vi "TestIniLib.vi"() -> ()   [LabVIEW 2014]
uses:
  <vilib>/Utility/config.llb/Config Data RefNum.ctl
  <vilib>/Utility/error.llb/Error Cluster From Error Code.vi
  <vilib>/ErrorRing/Error Ring.xnode
  <vilib>/Utility/config.llb/NI_LVConfig.lvlib
  <userlib>/NIST/NISTErrorLib/NISTErrorLib.lvlib
  Ini_lib.lvlib
panel:
  in  "btnStop":bool
  out "ErrorArray Out":errorcluster[](array[cluster])
  in  "Cluster 3":cluster{"This Array":dbl[]}={"This Array"=[1.0, 2.0, 3.0]}
  in  "Cluster 2":cluster{"This Boolean":bool, "That Path":path}
  in  "Cluster 1":cluster{"This String":string, "That Number":dbl}
  in  "Table 3":string[][](table)
  in  "Table 2":string[][](table)
  in  "Table 1":string[][](table)
  in  "Ring 3":u16(ring) items=["Mod3.Plugin1", "Mod3.Plugin2", "Mod3.Plugin3"]
  in  "Ring 2":u16(ring) items=["Mod2.Plugin1", "Mod2.Plugin2", "Mod2.Plugin3"]
  in  "Ring 1":u16(ring) items=["Mod1.Plugin1", "Mod1.Plugin2", "Mod1.Plugin3"]
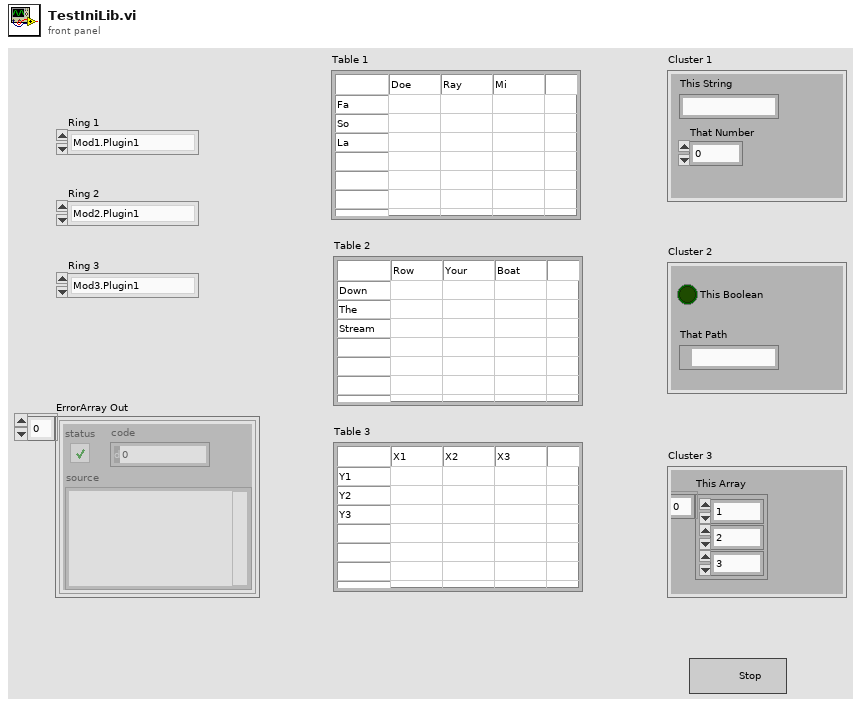
[diagram p1: front panel]
types:
  T1 = cluster{"Ring 1":refnum<vi>, "Table 1":refnum<vi>, "Cluster 1":refnum<vi>, "Ring 2":refnum<vi>, "Table 2":refnum<vi>, "Cluster 2":refnum<vi>, "Ring 3":refnum<vi>, "Table 3":refnum<vi>, "Cluster 3":refnum<vi>}
  T2 = typedef "NI_LVConfig.lvlib/Config Data RefNum.ctl" = refnum<k1>
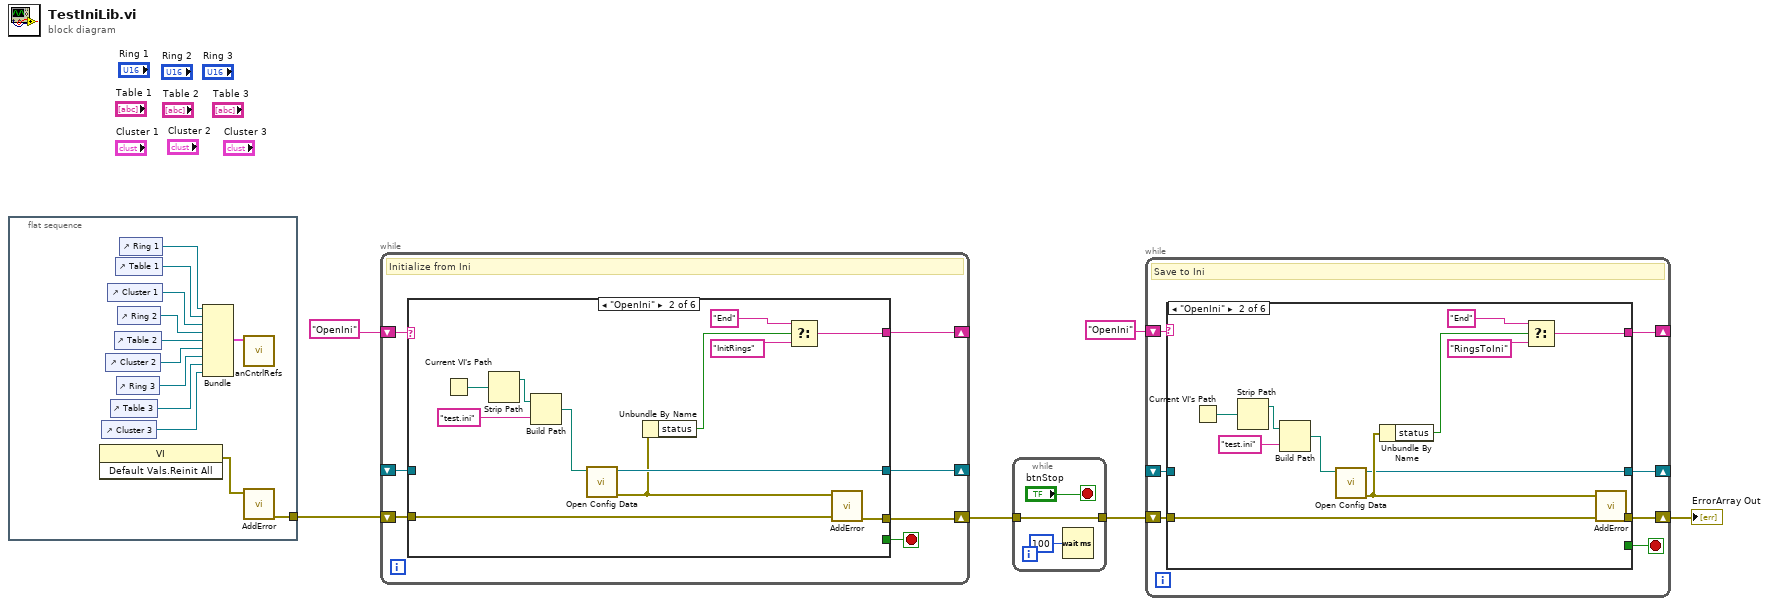
[diagram p0: block diagram]
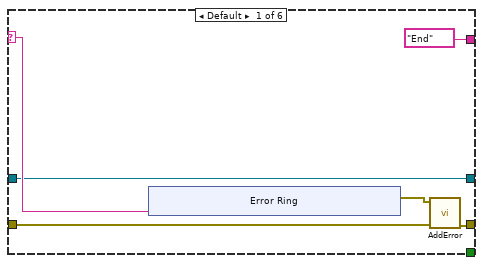
[diagram p2: hidden frame]
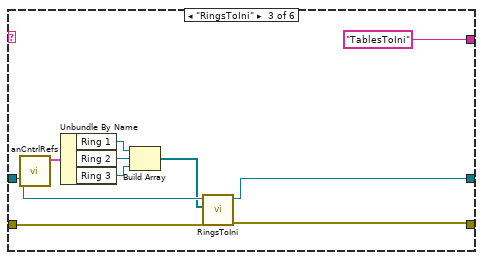
[diagram p3: hidden frame]
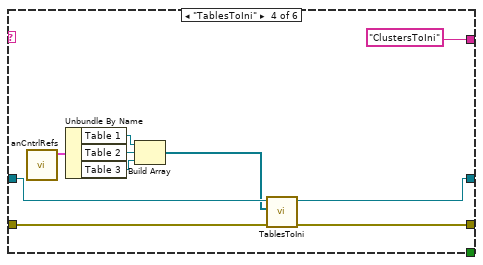
[diagram p4: hidden frame]
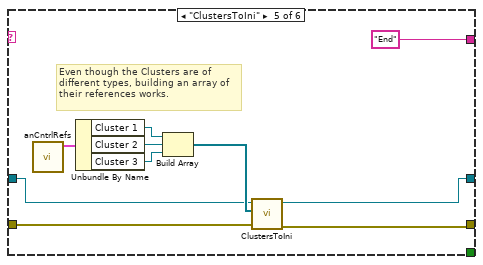
[diagram p5: hidden frame]
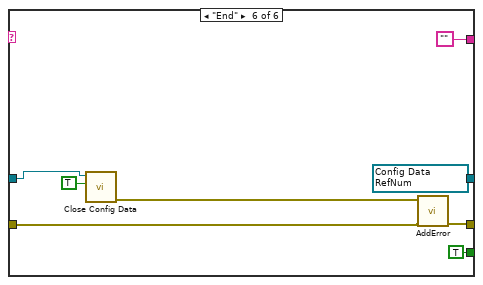
[diagram p6: hidden frame]
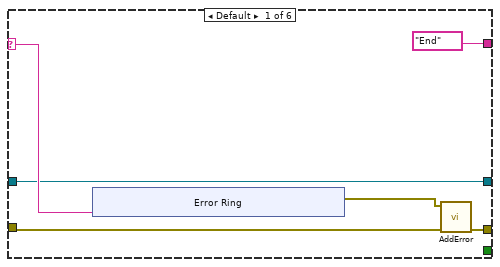
[diagram p7: hidden frame]
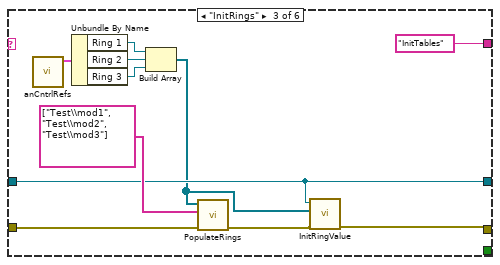
[diagram p8: hidden frame]
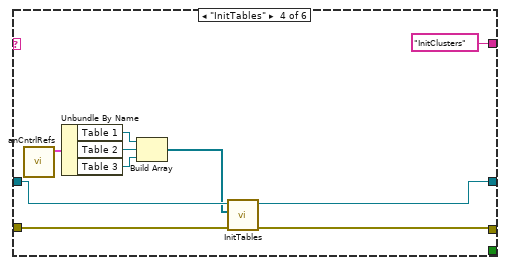
[diagram p9: hidden frame]
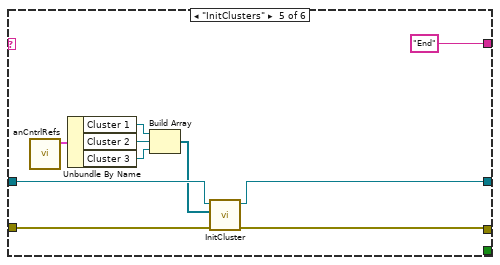
[diagram p10: hidden frame]
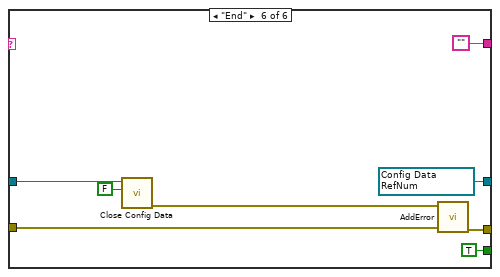
[diagram p11: hidden frame]
diagram:
  n1 = flat-sequence {
    tunnel: [w8] -> w6
    frame #0 {
      n2 = invoke class="VI" method="Default Vals.Reinit All"() -> (error out=w7:errorcluster)  [unwired: 3 in, 2 out]
      n3 = control-ref of="Cluster 3"() -> (w10:refnum<vi>)
      n4 = control-ref of="Cluster 2"() -> (w13:refnum<vi>)
      n5 = control-ref of="Cluster 1"() -> (w16:refnum<vi>)
      n6 = control-ref of="Table 3"() -> (w11:refnum<vi>)
      n7 = control-ref of="Table 2"() -> (w14:refnum<vi>)
      n8 = control-ref of="Table 1"() -> (w17:refnum<vi>)
      n9 = control-ref of="Ring 3"() -> (w12:refnum<vi>)
      n10 = control-ref of="Ring 2"() -> (w15:refnum<vi>)
      n11 = control-ref of="Ring 1"() -> (w18:refnum<vi>)
      n12 = Bundle("Ring 1"=w18, "Table 1"=w17, "Cluster 1"=w16, "Ring 2"=w15, "Table 2"=w14, "Cluster 2"=w13, "Ring 3"=w12, "Table 3"=w11, "Cluster 3"=w10) -> (w9:T1)  [unwired: 1 in]
      n13 = call "anCntrlRefs.vi"("CntrlRefs"=w9) -> ()  [unwired: 10 in, 1 out]
      n14 = call <userlib>:"AddError.vi"("error in (no error)"=w7) -> ("ErrorArray"=w8:errorcluster[])  [unwired: 9 in, 1 out]
    }
  }
  n15 = while {
    shift-right: [w24] -> _
    shift-left: _ -> [w21]
    shift-right: [w22] -> _
    shift-left: "OpenIni" -> [w25]
    shift-right: [w19] -> w2
    shift-left: w6 -> [w23]
    stop <- w20 stop-if-true
    # "Initialize from Ini"
    n16 = case shown="\"OpenIni\"" w25 {
      selector: w25 -> [w28 _ _ _ _ _]
      tunnel: [w26 w48 w52 w67 w73 w82] -> w24
      tunnel: w23 -> [w30 w47 w61 w70 w76 w84]
      tunnel: [w31 w46 w53 w69 w75 w85] -> w19
      tunnel: ["End" w41 "InitTables" "InitClusters" "End" ""] -> w22
      tunnel: w21 -> [w26 _ w52 w68 w74 w87]
      tunnel: [_ _ _ _ _ TRUE] -> w20
      frame Default {
        n17 = xnode "Error Ring"("parameter 0"=w28) -> ("error out"=w29:errorcluster)
        n18 = call <userlib>:"AddError.vi"("ErrorArray"=w30, "error in (no error)"=w29) -> ("ErrorArray"=w31:errorcluster[])  [unwired: 8 in, 1 out]
      }
      frame "OpenIni" {
        n19 = Current VI's Path() -> (path=w39:path)
        n20 = Strip Path(path=w39) -> (stripped path=w40:path)  [unwired: 1 out]
        n21 = Build Path(base path=w40, name or relative path="test.ini") -> (appended path=w49:path)
        n22 = call <vilib>:"Open Config Data.vi"("configuration file path"=w49) -> ("error out"=w45:errorcluster, "refnum"=w48:T2)  [unwired: 8 in, 1 out]
        n23 = Unbundle By Name(w45) -> ("status"=w44:bool)
        n24 = Select(t="End", s=w44, f="InitRings") -> (s? t:f=w41:string)
        n25 = call <userlib>:"AddError.vi"("ErrorArray"=w47, "error in (no error)"=w45) -> ("ErrorArray"=w46:errorcluster[])  [unwired: 8 in, 1 out]
      }
      frame "InitRings" {
        n26 = call "anCntrlRefs.vi"() -> ("CntrlRefs"=w60:T1)  [unwired: 11 in]
        n27 = Unbundle By Name(w60) -> ("Ring 1"=w59:refnum<vi>, "Ring 2"=w58:refnum<vi>, "Ring 3"=w57:refnum<vi>)
        n28 = Build Array(w59, w58, w57) -> (w51:refnum<vi>[])
        n29 = call "PopulateRings.vi"("ErrorArray In"=w61, "RelativePathToIniArray"=string[] ["Test\\mod1", "Test\\mod2", "Test\\mod3"], "RingRefArray"=w51) -> ("ErrorArray Out"=w54:errorcluster[])  [unwired: 7 in, 1 out]
        n30 = call "InitRingValue.vi"("ErrorArray In"=w54, "RingRefArray"=w51, "IniFileRef"=w52) -> ("ErrorArray Out"=w53:errorcluster[])  [unwired: 7 in, 1 out]
      }
      frame "InitTables" {
        n31 = call "anCntrlRefs.vi"() -> ("CntrlRefs"=w66:T1)  [unwired: 11 in]
        n32 = Unbundle By Name(w66) -> ("Table 1"=w64:refnum<vi>, "Table 2"=w65:refnum<vi>, "Table 3"=w63:refnum<vi>)
        n33 = Build Array(w64, w65, w63) -> (w62:refnum<vi>[])
        n34 = call "InitTables.vi"("ErrorArray in"=w70, "TableRefArray"=w62, "IniFileRef in"=w68) -> ("ErrorArray Out"=w69:errorcluster[], "IniFileRef out"=w67:T2)  [unwired: 7 in]
      }
      frame "InitClusters" {
        n35 = call "anCntrlRefs.vi"() -> ("CntrlRefs"=w80:T1)  [unwired: 11 in]
        n36 = Unbundle By Name(w80) -> ("Cluster 1"=w79:refnum<vi>, "Cluster 2"=w78:refnum<vi>, "Cluster 3"=w77:refnum<vi>)
        n37 = Build Array(w79, w78, w77) -> (w72:refnum<vi>[])
        n38 = call "InitCluster.vi"("ErrorArray in"=w76, "ClusterRefArray"=w72, "IniFileRef in"=w74) -> ("ErrorArray Out"=w75:errorcluster[], "IniFileRef out"=w73:T2)  [unwired: 7 in]
      }
      frame "End" {
        w82 = T2 refnum items=["config data"] ("refnum")
        n39 = call <vilib>:"Close Config Data.vi"("write file if changed (T)"=FALSE, "refnum"=w87) -> ("error out"=w83:errorcluster)  [unwired: 8 in, 1 out]
        n40 = call <userlib>:"AddError.vi"("ErrorArray"=w84, "error in (no error)"=w83) -> ("ErrorArray"=w85:errorcluster[])  [unwired: 8 in, 1 out]
      }
    }
  }
  n41 = while {
    tunnel: w2 -> [w91]
    tunnel: [w91] -> w1
    stop <- "btnStop" stop-if-true
    n42 = Wait (ms)(milliseconds to wait=u32 100) -> ()  [unwired: 1 out]
  }
  n43 = while {
    shift-right: [w96] -> _
    shift-left: "OpenIni" -> [w97]
    shift-right: [w95] -> _
    shift-left: _ -> [w94]
    shift-right: [w98] -> w4
    shift-left: w1 -> [w99]
    stop <- w93 stop-if-true
    # "Save to Ini"
    n44 = case shown="\"OpenIni\"" w97 {
      selector: w97 -> [w102 _ _ _ _ _]
      tunnel: [w105 w120 w132 w142 w152 w160] -> w98
      tunnel: w99 -> [w103 w119 w134 w143 w153 w161]
      tunnel: ["End" w114 "TablesToIni" "ClustersToIni" "End" ""] -> w96
      tunnel: [w100 w113 w133 w140 w145 w156] -> w95
      tunnel: w94 -> [w100 _ w131 w141 w146 w158]
      tunnel: [_ _ _ _ _ TRUE] -> w93
      frame Default {
        n45 = xnode "Error Ring"("parameter 0"=w102) -> ("error out"=w104:errorcluster)
        n46 = call <userlib>:"AddError.vi"("ErrorArray"=w103, "error in (no error)"=w104) -> ("ErrorArray"=w105:errorcluster[])  [unwired: 8 in, 1 out]
      }
      frame "OpenIni" {
        n47 = Current VI's Path() -> (path=w124:path)
        n48 = Strip Path(path=w124) -> (stripped path=w123:path)  [unwired: 1 out]
        n49 = Build Path(base path=w123, name or relative path="test.ini") -> (appended path=w121:path)
        n50 = call <vilib>:"Open Config Data.vi"("configuration file path"=w121) -> ("error out"=w115:errorcluster, "refnum"=w113:T2)  [unwired: 8 in, 1 out]
        n51 = Unbundle By Name(w115) -> ("status"=w116:bool)
        n52 = Select(t="End", s=w116, f="RingsToIni") -> (s? t:f=w114:string)
        n53 = call <userlib>:"AddError.vi"("ErrorArray"=w119, "error in (no error)"=w115) -> ("ErrorArray"=w120:errorcluster[])  [unwired: 8 in, 1 out]
      }
      frame "RingsToIni" {
        n54 = call "anCntrlRefs.vi"() -> ("CntrlRefs"=w130:T1)  [unwired: 11 in]
        n55 = Unbundle By Name(w130) -> ("Ring 1"=w127:refnum<vi>, "Ring 2"=w129:refnum<vi>, "Ring 3"=w128:refnum<vi>)
        n56 = Build Array(w127, w129, w128) -> (w126:refnum<vi>[])
        n57 = call "RingsToIni.vi"("ErrorArray in"=w134, "RingRefArray"=w126, "IniFileRef in"=w131) -> ("ErrorArray out"=w132:errorcluster[], "InifileRef out"=w133:T2)  [unwired: 7 in]
      }
      frame "TablesToIni" {
        n58 = call "anCntrlRefs.vi"() -> ("CntrlRefs"=w139:T1)  [unwired: 11 in]
        n59 = Unbundle By Name(w139) -> ("Table 1"=w138:refnum<vi>, "Table 2"=w137:refnum<vi>, "Table 3"=w136:refnum<vi>)
        n60 = Build Array(w138, w137, w136) -> (w135:refnum<vi>[])
        n61 = call "TablesToIni.vi"("ErrorArray in"=w143, "TableRefArray"=w135, "IniFileRef in"=w141) -> ("ErrorArray out"=w142:errorcluster[], "IniFileRef out"=w140:T2)  [unwired: 7 in]
      }
      frame "ClustersToIni" {
        # "Even though the Clusters are of different types, building an array of their references works."
        n62 = call "anCntrlRefs.vi"() -> ("CntrlRefs"=w151:T1)  [unwired: 11 in]
        n63 = Unbundle By Name(w151) -> ("Cluster 1"=w150:refnum<vi>, "Cluster 2"=w149:refnum<vi>, "Cluster 3"=w148:refnum<vi>)
        n64 = Build Array(w150, w149, w148) -> (w147:refnum<vi>[])
        n65 = call "ClustersToIni.vi"("ErrorArray in"=w153, "ClusterRefArray"=w147, "IniFileRef in"=w146) -> ("ErrorArray out"=w152:errorcluster[], "IniFileRef out"=w145:T2)  [unwired: 7 in]
      }
      frame "End" {
        w156 = T2 refnum items=["config data"] ("InifileRef out")
        n66 = call <vilib>:"Close Config Data.vi"("write file if changed (T)"=TRUE, "refnum"=w158) -> ("error out"=w159:errorcluster)  [unwired: 8 in, 1 out]
        n67 = call <userlib>:"AddError.vi"("ErrorArray"=w161, "error in (no error)"=w159) -> ("ErrorArray"=w160:errorcluster[])  [unwired: 8 in, 1 out]
      }
    }
  }
  "ErrorArray Out" <- w4
